vi "Connect OPC UA.vi"(6 "Sequence Context":refnum<k7>, 7 "OPC Ref Name":string="PLC Ref", 8 "error in":errorcluster, 9 "Trial Number":i32=3, 10 "timeout(s)":T2=5000, 11 "URL":string="opc.tcp://DESKTOP-T6QR0HI:4991/LunarTester") -> (0 "error out":errorcluster={"status"=TRUE, "code"=-356641, "source"="NI OPC UA Client.lvlib:Connect.vi"})   [LabVIEW 2021, in "OPCUA.lvlib"]
uses:
  <vilib>/OPCUA/controls/Time Out.ctl
  OPCUA.lvlib
  <vilib>/OPCUA/NI OPC UA Client.lvlib
panel:
  out "Note":string
  out "Waiting Lights":T1={"wait 1"=FALSE, "wait 2"=FALSE, "wait 3"=FALSE, "wait 4"=FALSE, "wait 5"=FALSE, "wait 6"=TRUE}
  out "Trial":i32=3
  out "stop":bool=TRUE
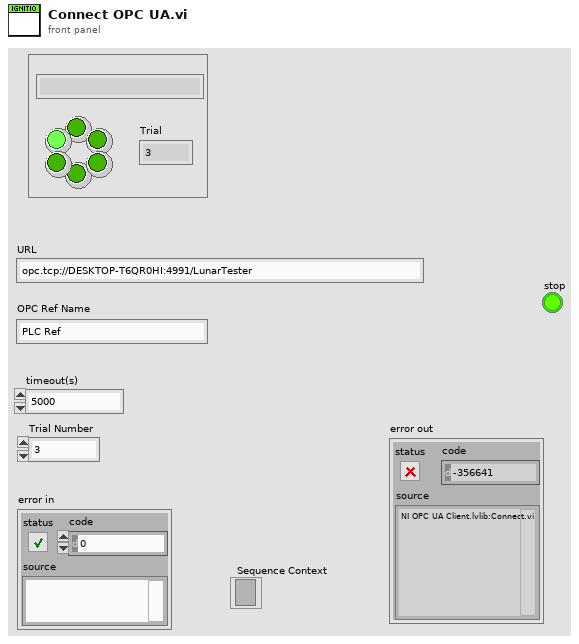
[diagram p1: front panel]
types:
  T1 = cluster{"wait 1":bool, "wait 2":bool, "wait 3":bool, "wait 4":bool, "wait 5":bool, "wait 6":bool}
  T2 = typedef "Time Out.ctl" = u32
  T3 = typedef "TestStand - Status Monitor.ctl" = cluster{"Sequence Context":refnum<k7>, "Execution":refnum<k7>, "Termination Monitor":refnum<k7>}
  T4 = typedef "OPC UA Client Refnum.ctl" = refnum<k21>
  T5 = cluster{"[0]":bool, "[1]":bool, "[2]":bool, "[3]":bool, "[4]":bool, "[5]":bool}
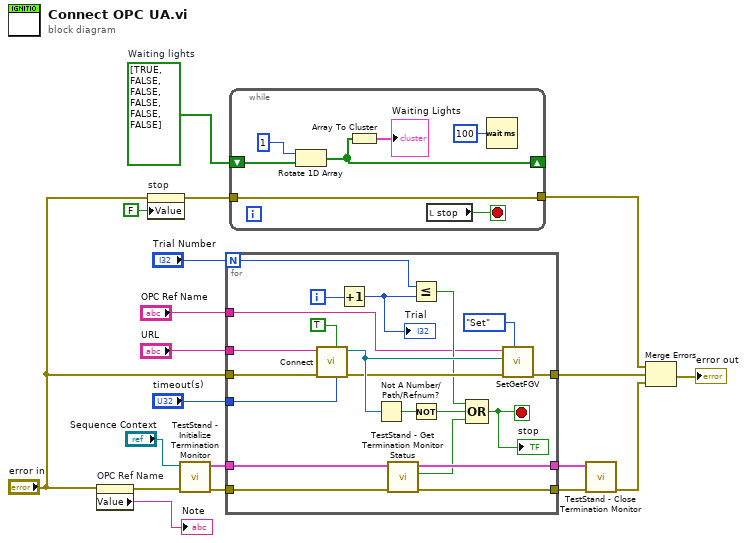
[diagram p0: block diagram]
diagram:
  w8 = bool[] [TRUE, FALSE, FALSE, FALSE, FALSE, FALSE]  # Waiting lights
  n1 = property on="OPC Ref Name" class="Str"(error in="error in") -> (error out=w1:errorcluster, "Value"=→"Note":string)  [unwired: 1 in, 1 out]
  n2 = property on="stop" class="Bool (strict)"(error in="error in", "Value"=FALSE ("stop")) -> (error out=w7:errorcluster)  [unwired: 1 in, 1 out]
  n3 = call <vilib>:"TestStand - Initialize Termination Monitor.vi"("error in (no error)"=w1, "Sequence Context In"="Sequence Context") -> ("error out"=w12:errorcluster, "Status Monitor Out"=w13:T3)  [unwired: 8 in]
  n4 = for {
    N: "Trial Number" -> [w26]
    tunnel: "URL" -> [w38]
    tunnel: w12 -> [w34]
    tunnel: w13 -> [w35]
    tunnel: [w33] -> w14
    tunnel: [w32] -> w16
    tunnel: "timeout(s)" -> [w20]
    tunnel: "OPC Ref Name" -> [w22]
    tunnel: "error in" -> [w39]
    tunnel: [w31] -> w15
    i -> [w30]
    stop <- w21 stop-if-true
    n5 = call <vilib>:"Connect.vi"("timeout (5000 ms)"=w20, "trust any server (F)"=TRUE, "error in (no error)"=w39, "server endpoint URL"=w38) -> ("error out"=w28:errorcluster, "OPC UA client refnum out"=w36:T4)  [unwired: 5 in, 1 out]
    n6 = Increment(x=w30) -> (x+1=w29:i32)
    "Trial" <- w29
    n7 = Not A Number/Path/Refnum?(number/path/refnum=w36) -> (NaN/Path/Refnum?=w27:bool)
    n8 = call <vilib>:"TestStand - Get Termination Monitor Status.vi"("error in (no error)"=w34, "Status Monitor In"=w35) -> ("error out"=w32:errorcluster, "Terminating or Aborting"=w23:bool, "Status Monitor Out"=w33:T3)  [unwired: 7 in]
    n9 = Less Or Equal?(x=w26, y=w29) -> (x <= y?=w24:bool)
    n10 = Not(x=w27) -> (.not. x?=w25:bool)
    n11 = Compound Arithmetic op=OR(w24, w25, w23) -> (w21:bool)
    "stop" <- w21
    n12 = call "SetGetFGV.vi"("Method (Get)"=enum16{"Get", "Set"}."Set", "error in"=w28, "Data In"=w36, "FGVname"=w22) -> ("error out"=w31:errorcluster)  [unwired: 6 in, 1 out]
  }
  n13 = while {
    tunnel: w7 -> [w45]
    tunnel: [w45] -> w6
    shift-right: [w42] -> _
    shift-left: w8 -> [w43]
    stop <- w46 stop-if-true
    n14 = Rotate 1D Array(1:w43, 2:1 ("n")) -> (0:w42:bool[])
    n15 = Array To Cluster(array=w42) -> (cluster=→"Waiting Lights":T5)
    n16 = local read "stop"() -> (w46:bool)
    n17 = Wait (ms)(milliseconds to wait=u32 100) -> ()  [unwired: 1 out]
  }
  n18 = call <vilib>:"TestStand - Close Termination Monitor.vi"("error in (no error)"=w16, "Status Monitor In"=w14) -> ("error out"=w17:errorcluster)  [unwired: 9 in]
  n19 = Merge Errors(w6, w15, w17) -> (→"error out":errorcluster)
